vi "ReceiveNorification.vi"(8 "error in (no error)":errorcluster, 11 "GeneralDisplay in":refnum<class "Dialog Notification.lvclass">) -> (0 "error out":errorcluster, 3 "GeneralDisplay out":refnum<class "Dialog Notification.lvclass">)   [LabVIEW 2020, in "Dialog Notification.lvclass"]
uses:
  Dialog Notification.lvclass
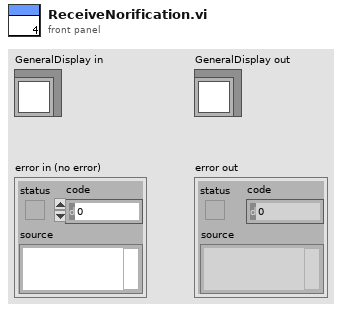
[diagram p1: front panel]
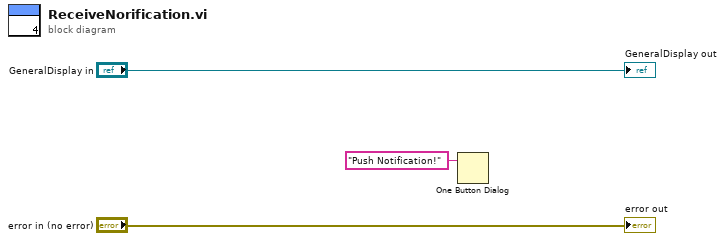
[diagram p0: block diagram]
diagram:
  n1 = One Button Dialog(message="Push Notification!") -> ()  [unwired: 1 in, 1 out]
  "error out" <- "error in (no error)"
  "GeneralDisplay out" <- "GeneralDisplay in"
